vi "Historico_consumo.vi"() -> ()   [LabVIEW 2024]
uses:
  DB_API/DB_API.lvclass
panel:
  out "Consumo":dbl[](graph)
  out "Hidrogeno":dynamicdata(graph)
  out "Presiones":dynamicdata(graph)
  out "error out":errorcluster
  out "body":string
  in  "IP":string
  out "concatenated string":string
  in  "fecha fin":timestamp
  in  "fecha inicio":timestamp
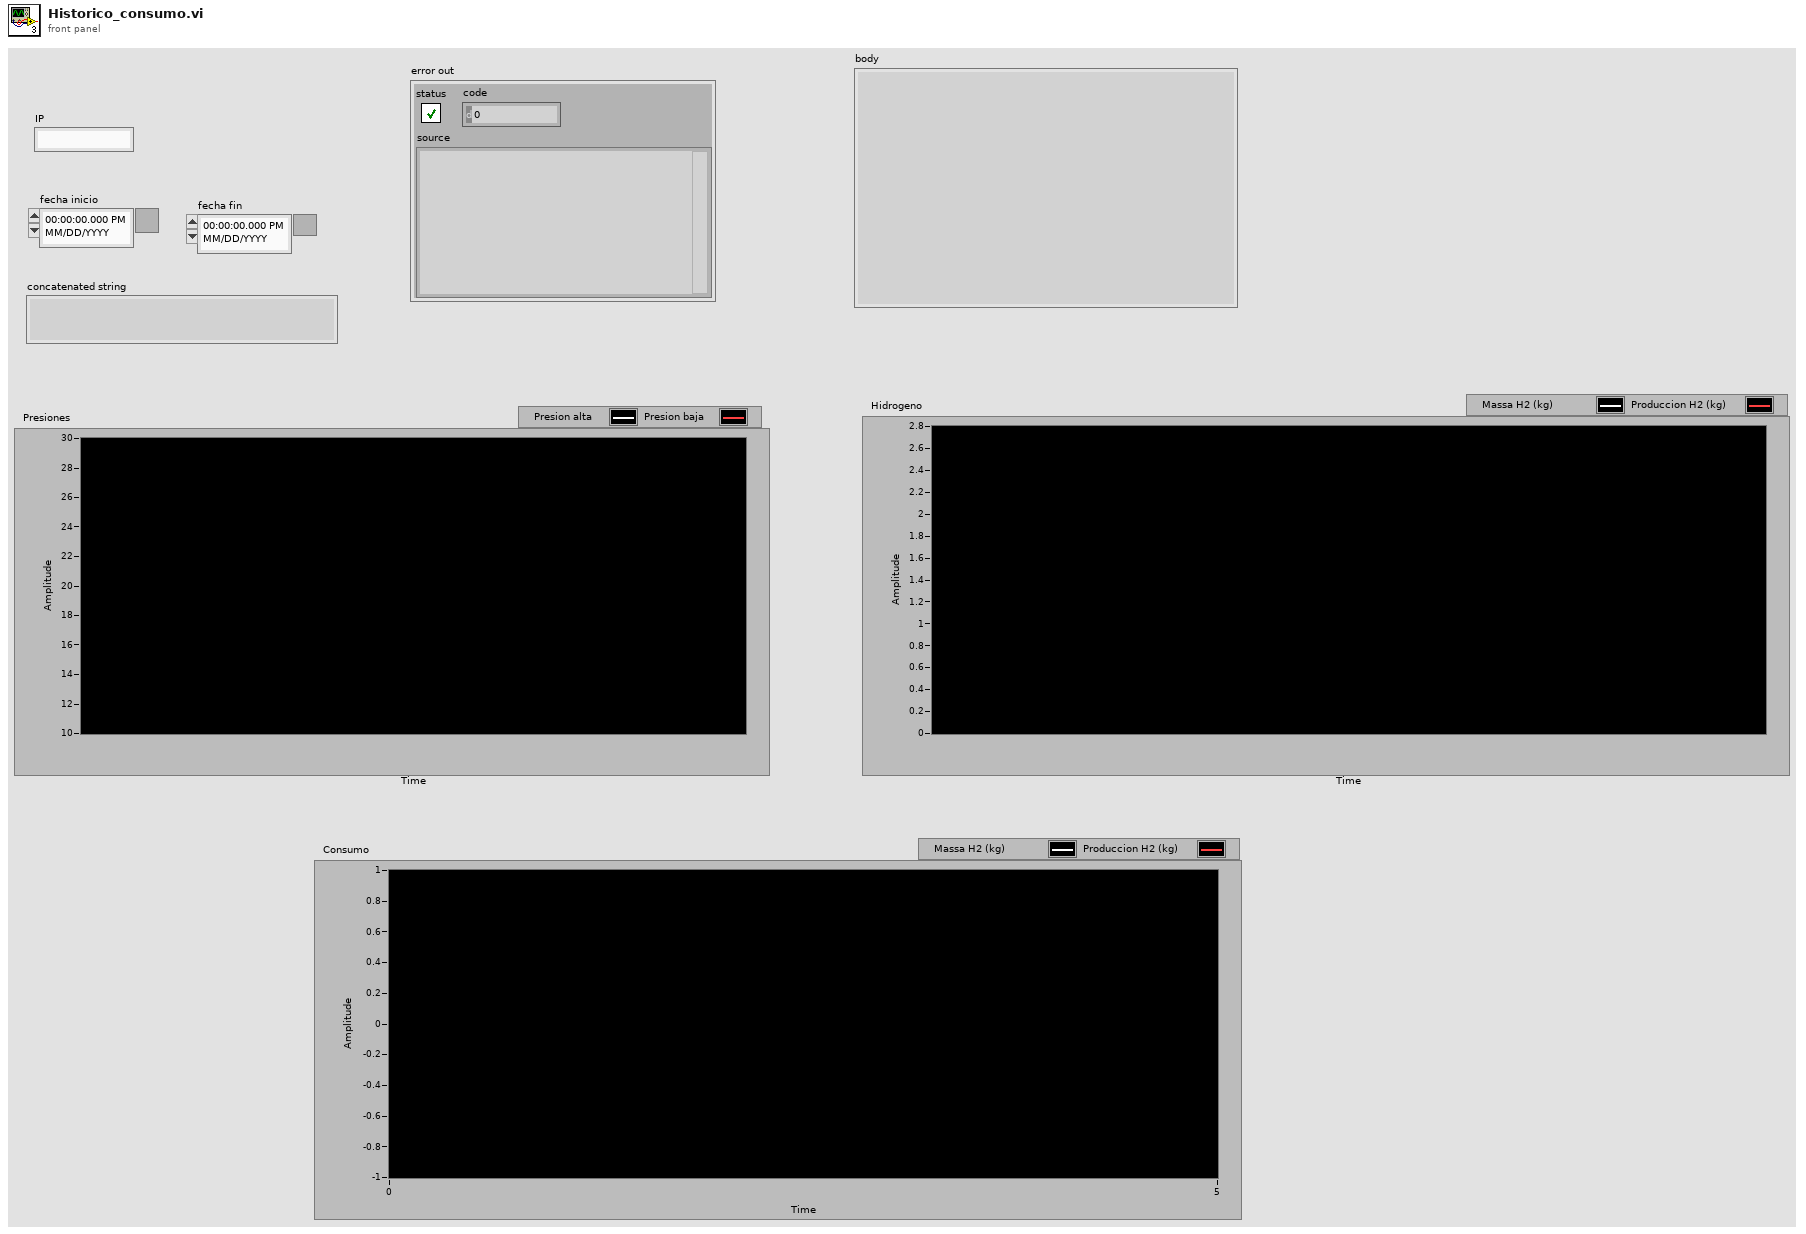
[diagram p1: front panel]
types:
  T1 = cluster{"fecha":string, "id":i32, "masa_alta":dbl, "masa_baja":dbl, "temperatura_exterior":dbl, "produccion_total":dbl, "presion_alta":dbl, "presion_baja":dbl}[]
  T2 = cluster{"fecha":string, "id":i32, "masa_alta":dbl, "masa_baja":dbl, "temperatura_exterior":dbl, "produccion_total":dbl, "presion_alta":dbl, "presion_baja":dbl}
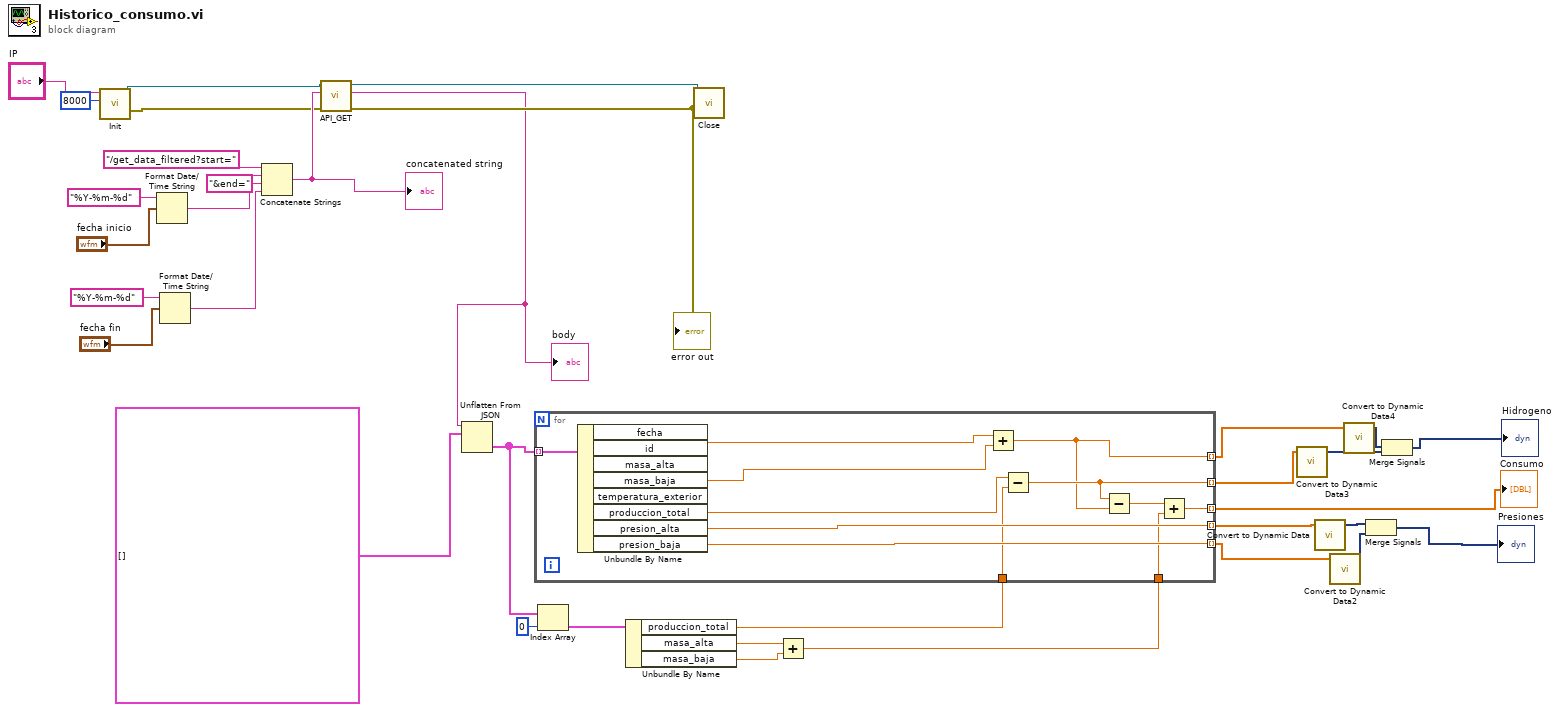
[diagram p0: block diagram]
diagram:
  n1 = call "Init.vi"("Port"=u32 8000, "IP"="IP") -> ("error out"=w25:errorcluster, "DB_API.lvclass 2"=w26:refnum<class "DB_API.lvclass">)  [unwired: 8 in]
  n2 = Format Date/Time String(time format string (%c)="%Y-%m-%d", seconds (now)="fecha inicio") -> (date/time string=w30:string)  [unwired: 1 in]
  n3 = Format Date/Time String(time format string (%c)="%Y-%m-%d", seconds (now)="fecha fin") -> (date/time string=w28:string)  [unwired: 1 in]
  n4 = Concatenate Strings("/get_data_filtered?start=" ("string"), w30, "&end=" ("string"), w28) -> (w27:string)
  "concatenated string" <- w27
  n5 = call "API_GET.vi"("error in (no error)"=w25, "endpoint"=w27, "DB_API.lvclass"=w26) -> ("error out"=w21:errorcluster, "body"=w20:string, "output cluster"=w22:refnum<class "DB_API.lvclass">)  [unwired: 4 in]
  "body" <- w20
  "error out" <- w21
  n6 = Unflatten From JSON(JSON string=w20, type and defaults=T1 []) -> (value=w9:T1)  [unwired: 5 in, 1 out]
  n7 = Index Array(array=w9, index=0) -> (element=w7:T2)
  n8 = Unbundle By Name(w7) -> ("produccion_total"=w6:dbl, "masa_alta"=w4:dbl, "masa_baja"=w3:dbl)
  n9 = call "Close.vi"("error in (no error)"=w21, "DB_API.lvclass 2"=w22) -> ()  [unwired: 9 in, 1 out]
  n10 = Add(x=w4, y=w3) -> (x+y=w2:dbl)
  n11 = for {
    tunnel: w9 -> [w47] mode=indexing
    tunnel: [w39] -> w12 mode=indexing
    tunnel: [w44] -> w17 mode=indexing
    tunnel: [w43] -> w15 mode=indexing
    tunnel: w6 -> [w41]
    tunnel: [w40] -> w5 mode=indexing
    tunnel: w2 -> [w37]
    tunnel: [w36] -> w1 mode=indexing
    n12 = Unbundle By Name(w47) -> ("masa_alta"=w46:dbl, "masa_baja"=w45:dbl, "produccion_total"=w42:dbl, "presion_alta"=w44:dbl, "presion_baja"=w43:dbl)  [unwired: 3 out]
    n13 = Add(x=w46, y=w45) -> (x+y=w39:dbl)
    n14 = Subtract(x=w42, y=w41) -> (x-y=w40:dbl)
    n15 = Subtract(x=w40, y=w39) -> (x-y=w38:dbl)
    n16 = Add(x=w38, y=w37) -> (x+y=w36:dbl)
  }
  "Consumo" <- w1
  n17 = call "Convert to Dynamic Data3"("Array"=w5) -> ("Dynamic Data Type"=w13:dynamicdata)  [unwired: 3 in]
  n18 = call "Convert to Dynamic Data"("Array"=w17) -> ("Dynamic Data Type"=w16:dynamicdata)  [unwired: 3 in]
  n19 = call "Convert to Dynamic Data2"("Array"=w15) -> ("Dynamic Data Type"=w14:dynamicdata)  [unwired: 3 in]
  n20 = call "Convert to Dynamic Data4"("Array"=w12) -> ("Dynamic Data Type"=w11:dynamicdata)  [unwired: 3 in]
  n21 = Merge Signals(w16, w14) -> (→"Presiones":dynamicdata)
  n22 = Merge Signals(w11, w13) -> (→"Hidrogeno":dynamicdata)
